vi "Get Repo Absolute Path.vi"() -> (3 "repo path":path)   [LabVIEW 2020]
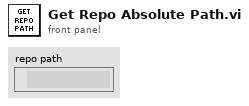
[diagram p1: front panel]
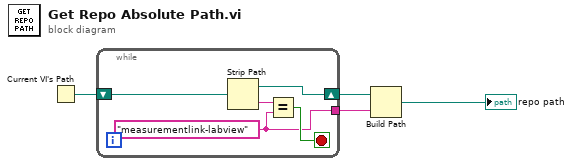
[diagram p0: block diagram]
diagram:
  n1 = Current VI's Path() -> (path=w2:path)
  n2 = while {
    shift-right: [w7] -> w3
    shift-left: w2 -> [w9]
    tunnel: [w5] -> w4
    stop <- w6 stop-if-true
    w5 = "measurementlink-labview" ("name")
    n3 = Strip Path(path=w9) -> (stripped path=w7:path, name=w8:string)
    n4 = Equal?(x=w8, y=w5) -> (x = y?=w6:bool)
  }
  n5 = Build Path(base path=w3, name or relative path=w4) -> (appended path=→"repo path":path)
